vi "proc_memory.vi"(11 "id":u32=5672) -> (0 "return":i32, 2 "info 2":u32[](array[numeric]))   [LabVIEW 2016]
uses:
  processHandles.dll
panel:
  in  "info":u32[](array[numeric])=[0, 0, 0, 0, 0, 0, 0, 0, 0, 0]
  # "DWORD cb;\n  DWORD PageFaultCount;\n  SIZE_T PeakWorkingSetSize;\n  SIZE_T WorkingSetSize;\n  SIZE_T QuotaPeakPagedPoolUsage;\n  SIZE_T QuotaPagedPoolUsage;\n  SIZE_T QuotaPeakNonPagedPoolUsage;\n  SIZE_T QuotaNonPagedPoolUsage;\n  SIZE_T PagefileUsage;\n  SIZE_T PeakPagefileUsage;"
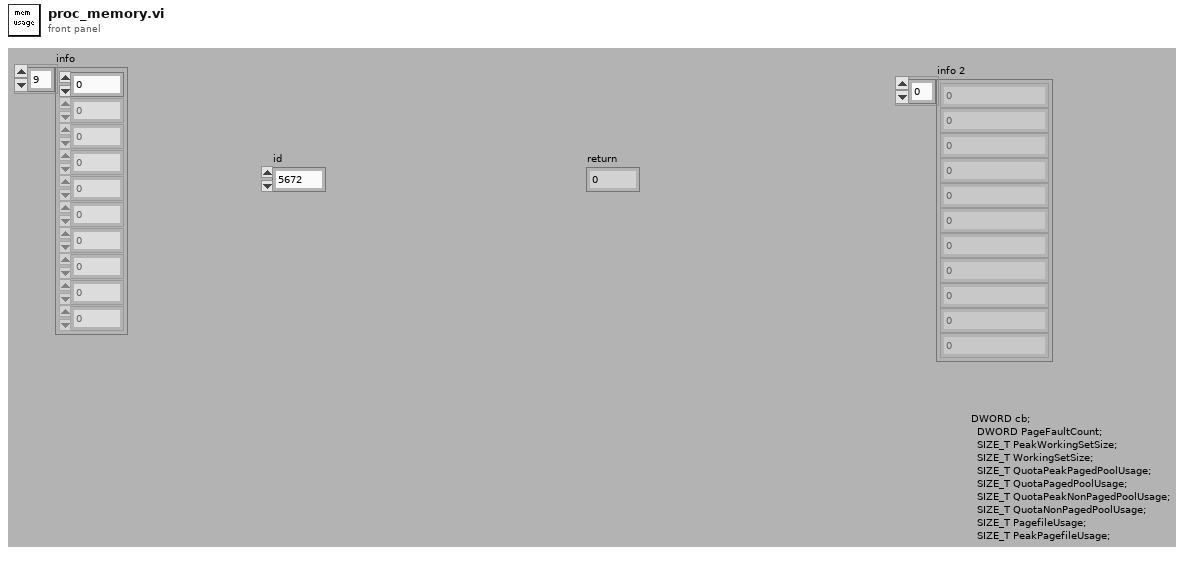
[diagram p1: front panel]
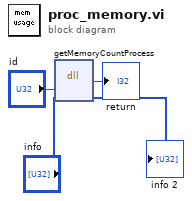
[diagram p0: block diagram]
diagram:
  n1 = dll-call lib="C:/Technology Lab/NI-2010/Trunk/Utility/Project Memory Manager/Project Manager/processHandles.dll" fn="getMemoryCountProcess"("id"="id", "info"="info") -> ("return type"=→"return":i32, "info"=→"info 2":u32[])  [unwired: 4 in, 2 out]
